vi "SelectMenuButtons.vi"(8 "error in":errorcluster, 11 "NewVal":T1) -> (0 "error out":errorcluster, 3 "Numeric":u32)   [LabVIEW 2016]
doc: "Retrun the number of the button press"
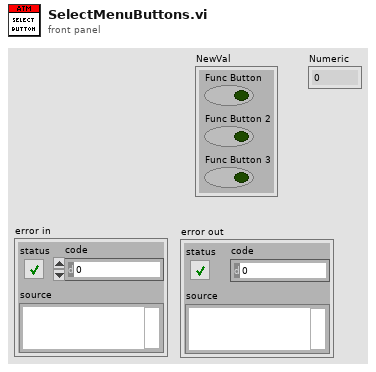
[diagram p1: front panel]
types:
  T1 = cluster{"Func Button":bool, "Func Button 2":bool, "Func Button 3":bool}
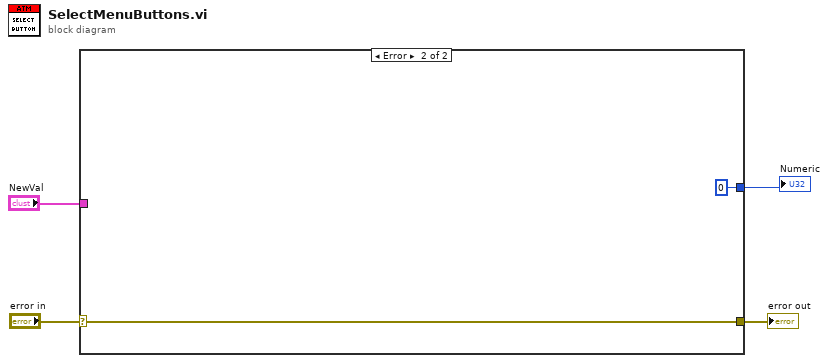
[diagram p0: block diagram]
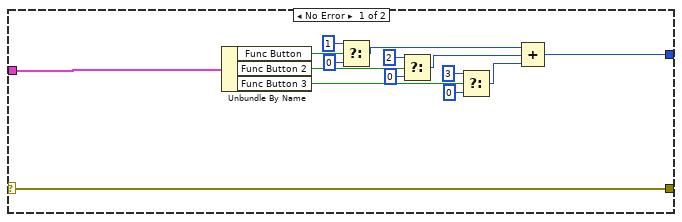
[diagram p2: hidden frame]
diagram:
  n1 = case shown="Error" "error in" {
    selector: "error in" -> [w7 w20]
    tunnel: [w7 w20] -> w3
    tunnel: "NewVal" -> [w6 _]
    tunnel: [w5 u32 0] -> w1
    frame No Error {
      n2 = Unbundle By Name(w6) -> ("Func Button"=w8:bool, "Func Button 2"=w13:bool, "Func Button 3"=w16:bool)
      n3 = Select(t=u32 1, s=w8, f=u32 0) -> (s? t:f=w17:u32)
      n4 = Select(t=u32 2, s=w13, f=u32 0) -> (s? t:f=w18:u32)
      n5 = Select(t=u32 3, s=w16, f=u32 0) -> (s? t:f=w19:u32)
      n6 = Compound Arithmetic op=ADD(w17, w18, w19) -> (w5:u32)
    }
    frame Error {
    }
  }
  "error out" <- w3
  "Numeric" <- w1
